vi "Test Calibration.vi"(8 "error in":errorcluster, 9 "Device":string, 10 "Cal Data":timestamp) -> (0 "error out":errorcluster)   [LabVIEW 2018, in "Configuration.lvlib" / "Configuration.lvclass"]
uses:
  Configuration.lvclass
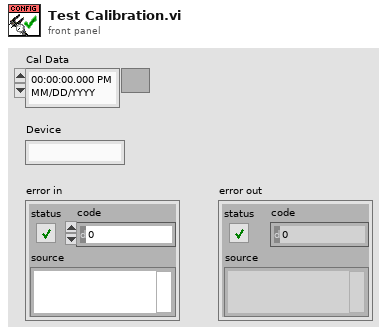
[diagram p1: front panel]
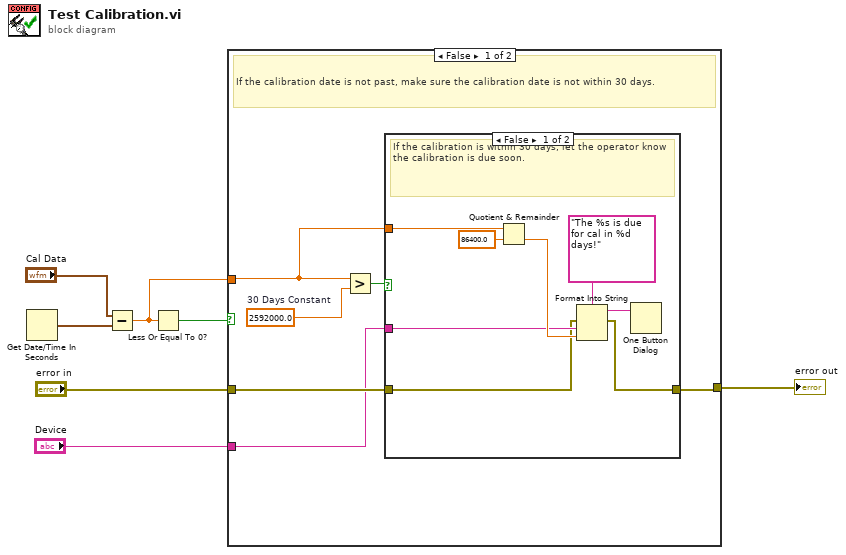
[diagram p0: block diagram]
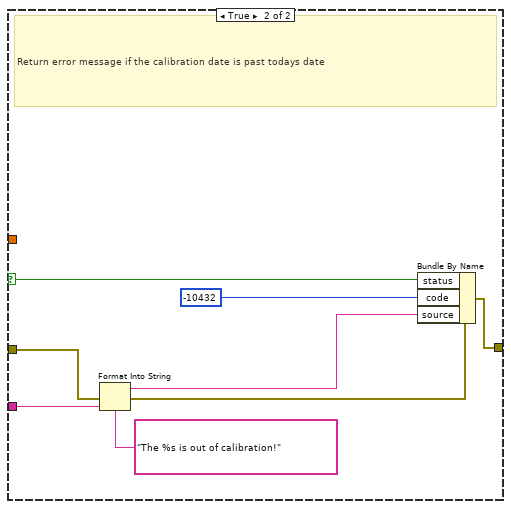
[diagram p3: hidden frame]
diagram:
  n1 = Get Date/Time In Seconds() -> (seconds since 1Jan1904=w6:timestamp)
  n2 = Subtract(x="Cal Data", y=w6) -> (x-y=w1:dbl)
  n3 = Less Or Equal To 0?(x=w1) -> (x <= 0?=w5:bool)
  n4 = case shown="False" w5 {
    selector: w5 -> [_ w29]
    tunnel: "error in" -> [w11 w26]
    tunnel: [w10 w30] -> w3
    tunnel: "Device" -> [w8 w27]
    tunnel: w1 -> [w9 _]
    frame False {
      w13 = 2592000.0  # 30 Days Constant
      # "If the calibration date is not past, make sure the calibration date is not within 30 days."
      n5 = Greater?(x=w9, y=w13) -> (0:w12:bool)
      n6 = case shown="False" w12 {
        tunnel: w11 -> [w15 w22]
        tunnel: [w14 w22] -> w10
        tunnel: w9 -> [w20 _]
        tunnel: w8 -> [w16 _]
        frame False {
          # "If the calibration is within 30 days, let the operator know the calibration is due soon."
          n7 = Quotient & Remainder(x=w20, y=86400.0) -> (floor(x/y)=w17:dbl)  [unwired: 1 out]
          n8 = Format Into String(format string="The %s is due for cal in %d days!", error in=w15, w16, w17) -> (resulting string=w21:string, error out=w14:errorcluster)  [unwired: 1 in]
          n9 = One Button Dialog(message=w21) -> ()  [unwired: 1 in, 1 out]
        }
        frame True {
          # "If the calibration date is further out than 30 days, return no error message."
        }
      }
    }
    frame True {
      # "Return error message if the calibration date is past todays date"
      n10 = Format Into String(format string="The %s is out of calibration!", error in=w26, w27) -> (resulting string=w24:string, error out=w25:errorcluster)  [unwired: 1 in]
      n11 = Bundle By Name(cluster=w25, "status"=w29, "code"=-10432, "source"=w24) -> (w30:errorcluster)
    }
  }
  "error out" <- w3
